vi "rs232test.vi"() -> ()   [LabVIEW 2010]
uses:
  <vilib>/Instr/_visa.llb/VISA Configure Serial Port (Instr).vi
panel:
  in  "stop":bool
  out "concatenated string":string
  out "error out":errorcluster
  in  "Send":bool
  in  "write buffer":string
  in  "VISA resource name":refnum<visa-resource-name>
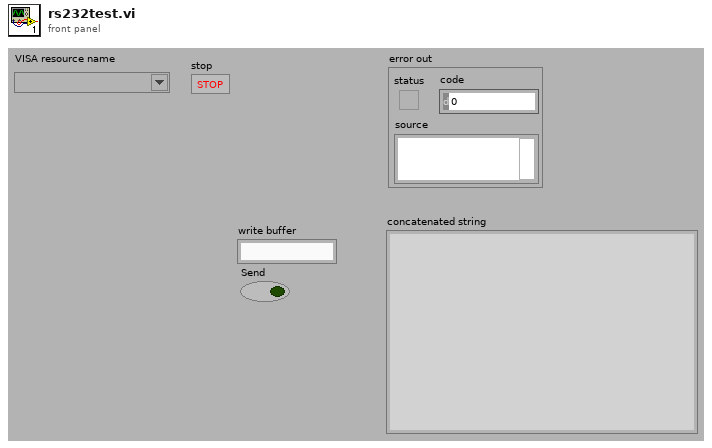
[diagram p1: front panel]
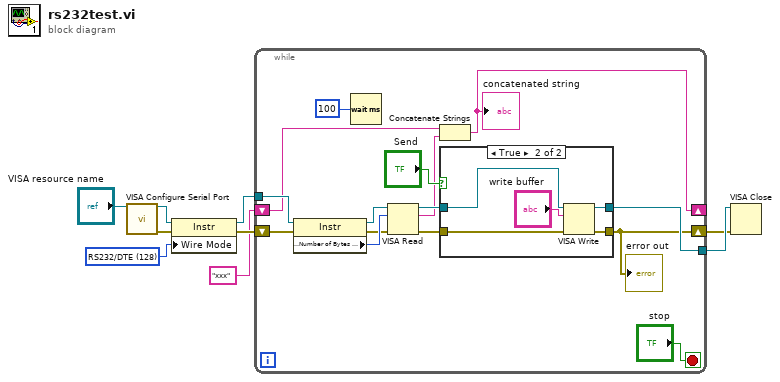
[diagram p0: block diagram]
diagram:
  w7 = i16 128 items=["Unknown"=-1, "RS485/Wire4"=0, "RS485/Wire2-EchoDTR"=1, "RS485/Wire2-CtrlDTR"=2, "RS485/Wire2-Auto"=3, "RS232/DTE"=128, "RS232/DCE"=129, "RS232/AUTO"=130] ("Serial Settings:Wire Mode")
  n1 = call-poly "VISA Configure Serial Port"("VISA resource name"="VISA resource name") -> ("VISA resource name out"=w8:refnum<visa-resource-name>, "error out"=w5:errorcluster)  [unwired: 13 in]
  n2 = property class="Instr"(reference=w8, error in=w5, "Wire Mode"=w7) -> (reference out=w6:refnum<visa-resource-name>, error out=w4:errorcluster)
  n3 = while {
    tunnel: w6 -> [w24]
    tunnel: [w20] -> w3
    shift-right: [w15] -> w2
    shift-left: w4 -> [w18]
    shift-right: [w11] -> _
    shift-left: "xxx" -> [w13]
    stop <- "stop" stop-if-true
    n4 = property class="Instr"(reference=w24, error in=w18) -> (reference out=w23:refnum<visa-resource-name>, error out=w17:errorcluster, "Serial Settings:Number of Bytes at Serial Port"=w22:u32)
    n5 = Wait (ms)(milliseconds to wait=u32 100) -> ()  [unwired: 1 out]
    n6 = VISA Read(VISA resource name=w23, byte count=w22, error in (no error)=w17) -> (VISA resource name out=w21:refnum<visa-resource-name>, read buffer=w12:string, error out=w16:errorcluster)  [unwired: 1 out]
    n7 = Concatenate Strings(w13, w12) -> (w11:string)
    "concatenated string" <- w11
    n8 = case shown="True" "Send" {
      tunnel: w21 -> [w26 w31]
      tunnel: [w26 w30] -> w20
      tunnel: w16 -> [w25 w28]
      tunnel: [w25 w27] -> w15
      frame False {
      }
      frame True {
        n9 = VISA Write(VISA resource name=w31, write buffer="write buffer", error in (no error)=w28) -> (VISA resource name out=w30:refnum<visa-resource-name>, error out=w27:errorcluster)  [unwired: 1 out]
      }
    }
    "error out" <- w15
  }
  n10 = VISA Close(VISA resource name=w3, error in (no error)=w2) -> ()  [unwired: 1 out]
